vi "GetVandBeishu.vi"() -> (1 "电压倍数":string, 2 "电压频率":string, 3 "输出电压值":string)   [LabVIEW 2014, in "DataBase.lvlib"]
uses:
  DataBase.lvlib
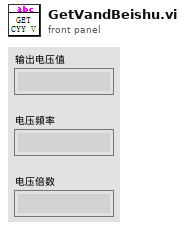
[diagram p1: front panel]
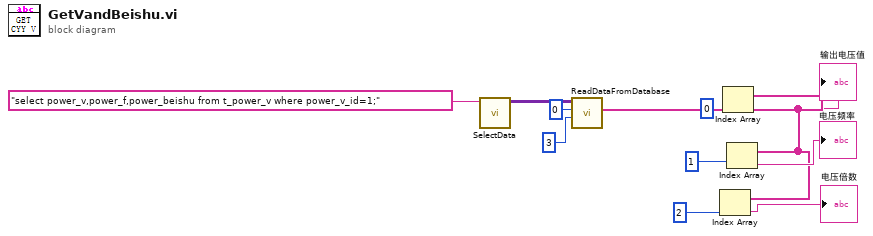
[diagram p0: block diagram]
diagram:
  n1 = call "SelectData.vi"("SQL query"="select power_v,power_f,power_beishu from t_power_v where power_v_id=1;") -> ("recordset data"=w2:variant[][])  [unwired: 7 in, 1 out]
  n2 = call "ReadDataFromDatabase.vi"("长度"=3, "index"=0, "recordset data"=w2) -> ("一行记录"=w8:string[])  [unwired: 7 in, 1 out]
  n3 = Index Array(array=w8, index=2) -> (element=→"电压倍数":string)
  n4 = Index Array(array=w8, index=0 ("索引")) -> (element=→"输出电压值":string)
  n5 = Index Array(array=w8, index=1) -> (element=→"电压频率":string)
